vi "ExpandData.vi"(8 "Data length":u8=1 min=1 max=2, 9 "Input":string) -> (2 "Output":i32[](array[numeric]))   [LabVIEW 2010]
doc: "Copyright (c) 2012 Metrolab Technology SA, Plan-les-Ouates, Geneva, Switzerland\nExpand compressed data. Only used as subVI for MEASure_FETCh_READ.vi."
panel:
  # "ExpandData"
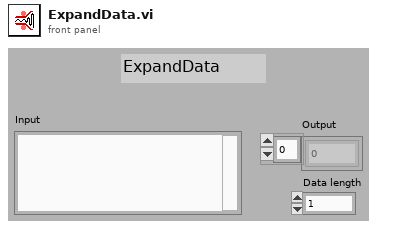
[diagram p1: front panel]
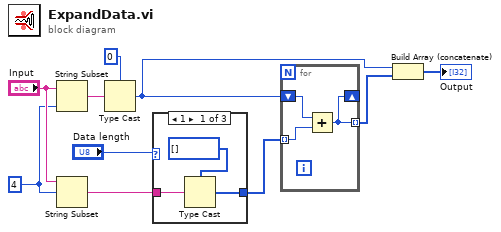
[diagram p0: block diagram]
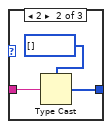
[diagram p2: hidden frame]
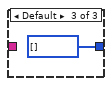
[diagram p3: hidden frame]
diagram:
  w4 = 4 ("offset (0)")
  n1 = String Subset(string="Input", length (rest)=w4) -> (substring=w8:string)  [unwired: 1 in]
  n2 = String Subset(string="Input", offset (0)=w4) -> (substring=w5:string)  [unwired: 1 in]
  n3 = Type Cast(type=0, x=w8) -> (*(type *) &x=w1:i32)
  n4 = case shown="1" "Data length" {
    tunnel: w5 -> [w11 w14 _]
    tunnel: [w12 w15 i16[] []] -> w7
    frame 1 {
      n5 = Type Cast(type=i8[] [], x=w11) -> (*(type *) &x=w12:i8[])
    }
    frame 2 {
      n6 = Type Cast(type=i16[] [], x=w14) -> (*(type *) &x=w15:i16[])
    }
    frame Default {
    }
  }
  n7 = for {
    tunnel: w7 -> [w18] mode=indexing
    shift-right: [w20] -> _
    shift-left: w1 -> [w19]
    tunnel: [w20] -> w2 mode=indexing
    n8 = Add(x=w19, y=w18) -> (x+y=w20:i32)
  }
  n9 = Build Array (concatenate)(w1, w2) -> (→"Output":i32[])
